vi "DD_Parameter.vi"() -> ()   [LabVIEW 2018, in "DataDisplay.lvlib"]
uses:
  DataDisplay.lvlib
  TypeDefine/DD_ChannelInfo.ctl
  TypeDefine/DD_DataStream.ctl
panel:
  in  "原始采样率":i32
  in  "DD_通道名称列表":string[](array[string])
  out "DD_数据通知器":refnum<notifier>
  in  "DD_采样率":i32
  out "DD_通道信息":T1[](array[typedef])
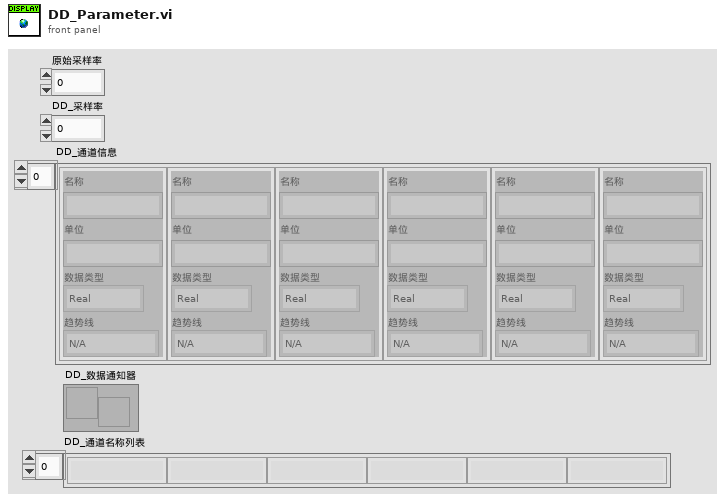
[diagram p1: front panel]
types:
  T1 = typedef "DataDisplay.lvlib/DD_ChannelInfo.ctl" = cluster{"名称":string, "单位":string, "数据类型":enum16{"Real", "Int"}, "趋势线":enum16{"N/A", "X", "Y"}}
diagram:
